vi "EventsLog Ref(FGV).vi"(8 "Error In":errorcluster, 9 "State":enum16{"Get", "Set"}(ring), 11 "EventLog In":refnum<class "EventLog.lvclass">) -> (0 "Error Out":errorcluster, 3 "EventLog Out":refnum<class "EventLog.lvclass">)   [LabVIEW 2019, in "EventLog.lvclass"]
uses:
  EventLog.lvclass
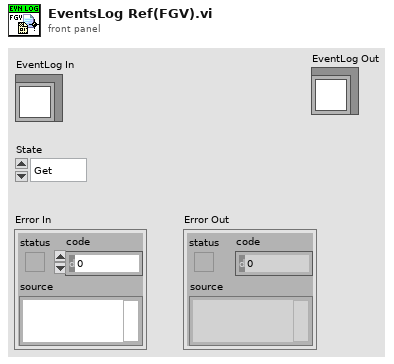
[diagram p1: front panel]
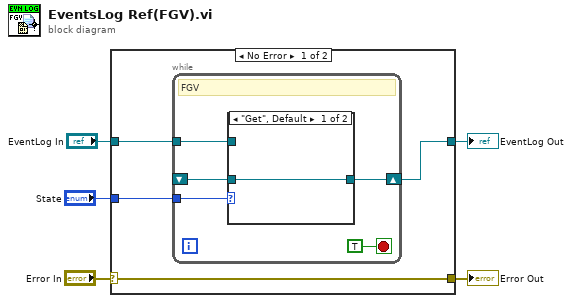
[diagram p0: block diagram]
diagram:
  n1 = case shown="No Error" "Error In" {
    selector: "Error In" -> [w9 w17]
    tunnel: [w9 w17] -> w4
    tunnel: "EventLog In" -> [w6 _]
    tunnel: [w8 _] -> w1
    tunnel: "State" -> [w7 _]
    frame No Error {
      n2 = while {
        tunnel: w7 -> [w13]
        tunnel: w6 -> [w12]
        shift-right: [w11] -> w8
        shift-left: _ -> [w10]
        stop <- TRUE stop-if-true
        # "FGV"
        n3 = case shown="\"Get\", Default" w13 {
          tunnel: w12 -> [_ w16]
          tunnel: [w15 w16] -> w11
          tunnel: w10 -> [w15 _]
          frame "Get", Default {
          }
          frame "Set" {
          }
        }
      }
    }
    frame Error {
    }
  }
  "Error Out" <- w4
  "EventLog Out" <- w1
